vi "AB_820_850_Project_Source.vi"(6 "dataForPrevious":T1, 7 "action":T7, 8 "error in (no error)":errorcluster, 9 "index in":i32, 10 "dataSource in":T6, 11 "buildObject":T4) -> (0 "error out":errorcluster, 1 "index out":i32, 2 "dataSource out":T6, 3 "buildObject out":T4)   [LabVIEW 2020]
doc: "Reads and writes the data to the object property bag."
uses:
  <resource>/Framework/Providers/API/ItemRef.ctl
  <vilib>/AppBuilder/AB_Source_Inclusion.ctl
  <vilib>/AppBuilder/RW_Project/AB_RW_Project_PropBag_Action.ctl
  <vilib>/AppBuilder/RW_Project/AB_RW_Project_Source_Data_for_Previous.ctl
  <vilib>/AppBuilder/AB_BuildType.ctl
  <vilib>/Utility/lvfile.llb/LVFileType.ctl
  <vilib>/AppBuilder/AB_Source_Property_WindowBehavior.ctl
  <vilib>/Utility/lvfile.llb/NI_FileType.lvlib
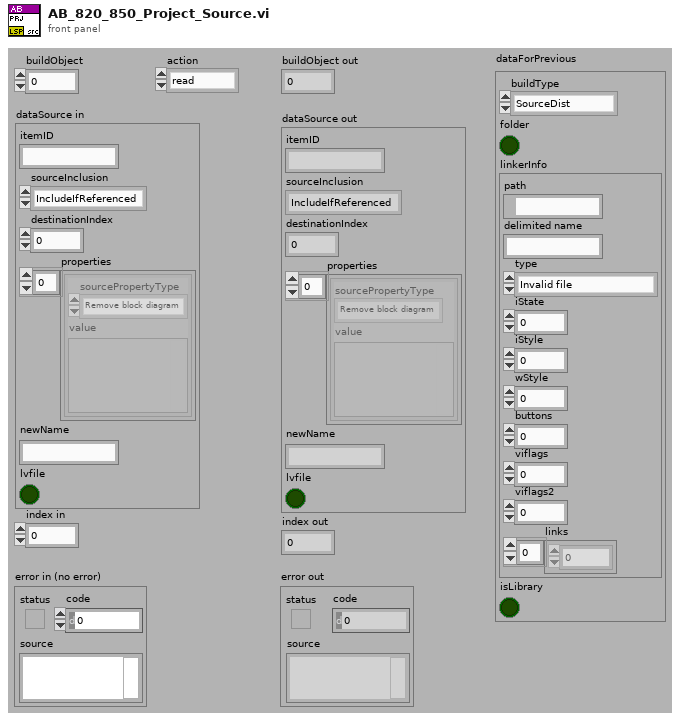
[diagram p1: front panel]
types:
  T1 = typedef "AB_RW_Project_Source_Data_for_Previous.ctl" = cluster{"buildType":T2, "folder":bool, "linkerInfo":cluster{"path":path, "delimited name":string, "type":T3, "iState":u32, "iStyle":u16, "wStyle":u16, "buttons":u16, "viflags":u32, "viflags2":u32, "links":u32[]}, "isLibrary":bool}
  T2 = typedef "AB_BuildType.ctl" = enum16{"SourceDist", "EXE", "DLL", "RTExe"}
  T3 = typedef "NI_FileType.lvlib/LVFileType.ctl" = enum32{"Invalid file", "Unknown type", "Instrument", "Control", "Polymorphic VI", "Project", "Library", "LVClass", "XControl", "XNode", "Shared library", ".NET assembly", "ActiveX interface", "CIN", "Run-time menu", "Palette menu", "Help file", "LLB", "XNode Edit Dependency", "Class Private Data Control", "Statechart", "MathScript .m file", "Ladder Diagram", "LVLibp", "XNode Build Dependency"}
  T4 = typedef "ItemRef.ctl" = u64
  T5 = typedef "AB_Source_Inclusion.ctl" = enum16{"IncludeIfReferenced", "Include", "Exclude", "TopLevel"}
  T6 = cluster{"itemID":string, "sourceInclusion":T5, "destinationIndex":i32, "properties":cluster{"sourcePropertyType":enum16{"Remove block diagram", "Remove front panel", "Password", "Window has title bar", "Show menu bar", "Show vertical scroll bar", "Show horizontal scroll bar", "Show toolbar", "Show Abort button", "Show fp when called", "Window behavior", "Allow user to close window", "Window run-time position", "Run when opened", "Allow debugging", "Auto error handling"}, "value":variant}[], "newName":string, "lvfile":bool}
  T7 = typedef "AB_RW_Project_PropBag_Action.ctl" = enum16{"read", "write", "clear", "readPrevious", "writePrevious", "clearPrevious"}
  T8 = cluster{"sourcePropertyType":enum16{"Remove block diagram", "Remove front panel", "Password", "Window has title bar", "Show menu bar", "Show vertical scroll bar", "Show horizontal scroll bar", "Show toolbar", "Show Abort button", "Show fp when called", "Window behavior", "Allow user to close window", "Window run-time position", "Run when opened", "Allow debugging", "Auto error handling"}, "value":variant}
  T9 = typedef "AB_Source_Property_WindowBehavior.ctl" = enum16{"Default", "Floating", "Modal"}
  T10 = cluster{"sourcePropertyType":enum16{"Remove block diagram", "Remove front panel", "Password", "Window has title bar", "Show menu bar", "Show vertical scroll bar", "Show horizontal scroll bar", "Show toolbar", "Show Abort button", "Show fp when called", "Window behavior", "Allow user to close window", "Window run-time position", "Run when opened", "Allow debugging", "Auto error handling"}, "value":variant}[]
  T11 = enum16{"Remove block diagram", "Remove front panel", "Password", "Window has title bar", "Show menu bar", "Show vertical scroll bar", "Show horizontal scroll bar", "Show toolbar", "Show Abort button", "Show fp when called", "Window behavior", "Allow user to close window", "Window run-time position", "Run when opened", "Allow debugging", "Auto error handling"}
  T12 = enum16{"Remove debugging", "Remove diagram", "Remove panel", "Show panel when called", "Run when opened", "Show abort button", "Window is modal", "Allow user to close window", "Window has title bar", "Show menu bar", "Show tool bar when running", "Show scroll bars", "Auto-center", "Size to entire screen", "Automatic error handling"}
  T13 = cluster{"applyInclusion":bool, "applyDestination":bool, "applyProperties":bool, "applyPassword":bool, "applyPrefix":bool, "applySaveSetttings":bool}
  T14 = cluster{"sourcePropertyType":enum16{"Remove block diagram", "Remove front panel", "Password", "Window has title bar", "Show menu bar", "Show vertical scroll bar", "Show horizontal scroll bar", "Show toolbar", "Show Abort button", "Show fp when called", "Window behavior", "Allow user to close window", "Window run-time position", "Run when opened", "Allow debugging", "Auto error handling"}, "Value":string}
  T15 = cluster{"sourcePropertyType":enum16{"Remove block diagram", "Remove front panel", "Password", "Window has title bar", "Show menu bar", "Show vertical scroll bar", "Show horizontal scroll bar", "Show toolbar", "Show Abort button", "Show fp when called", "Window behavior", "Allow user to close window", "Window run-time position", "Run when opened", "Allow debugging", "Auto error handling"}, string}
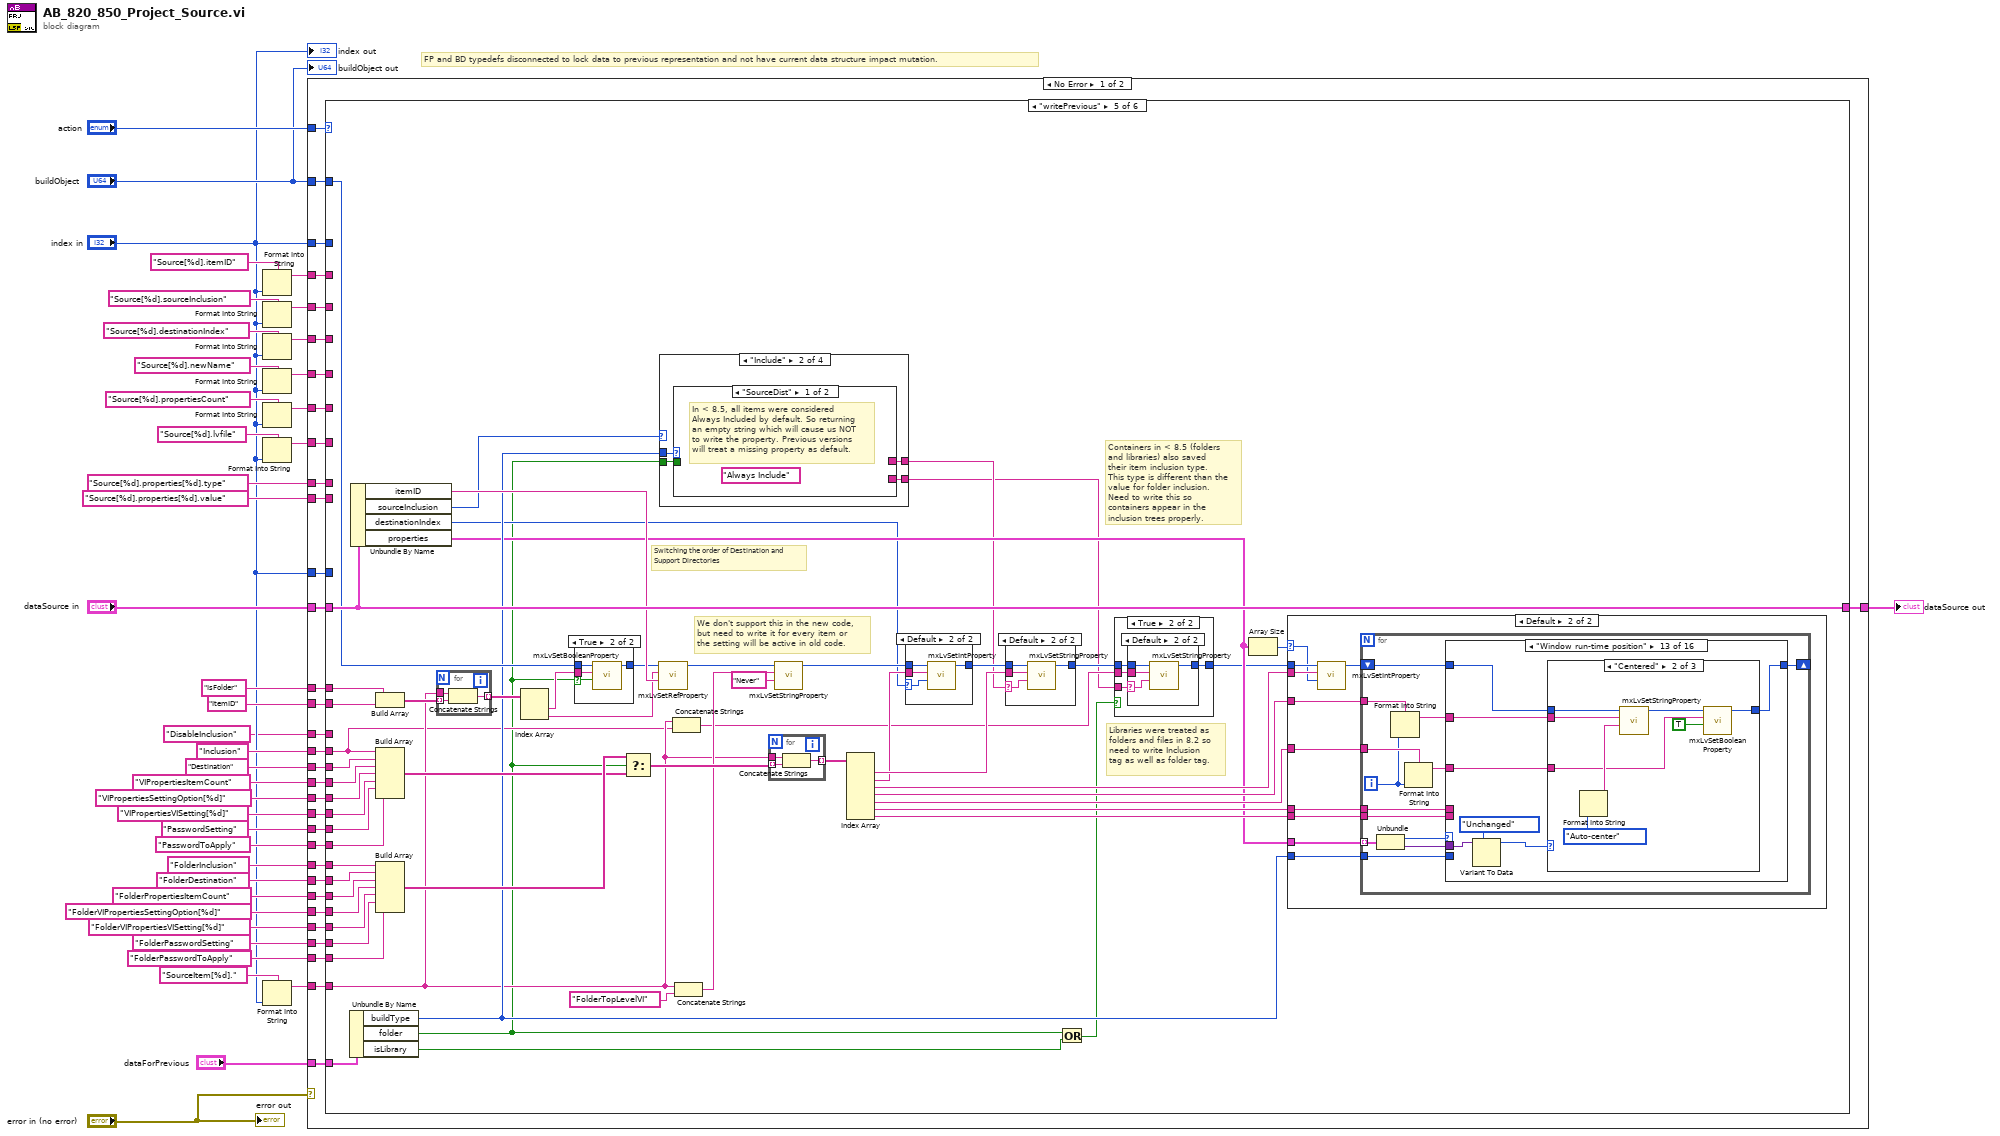
[diagram p0: block diagram]
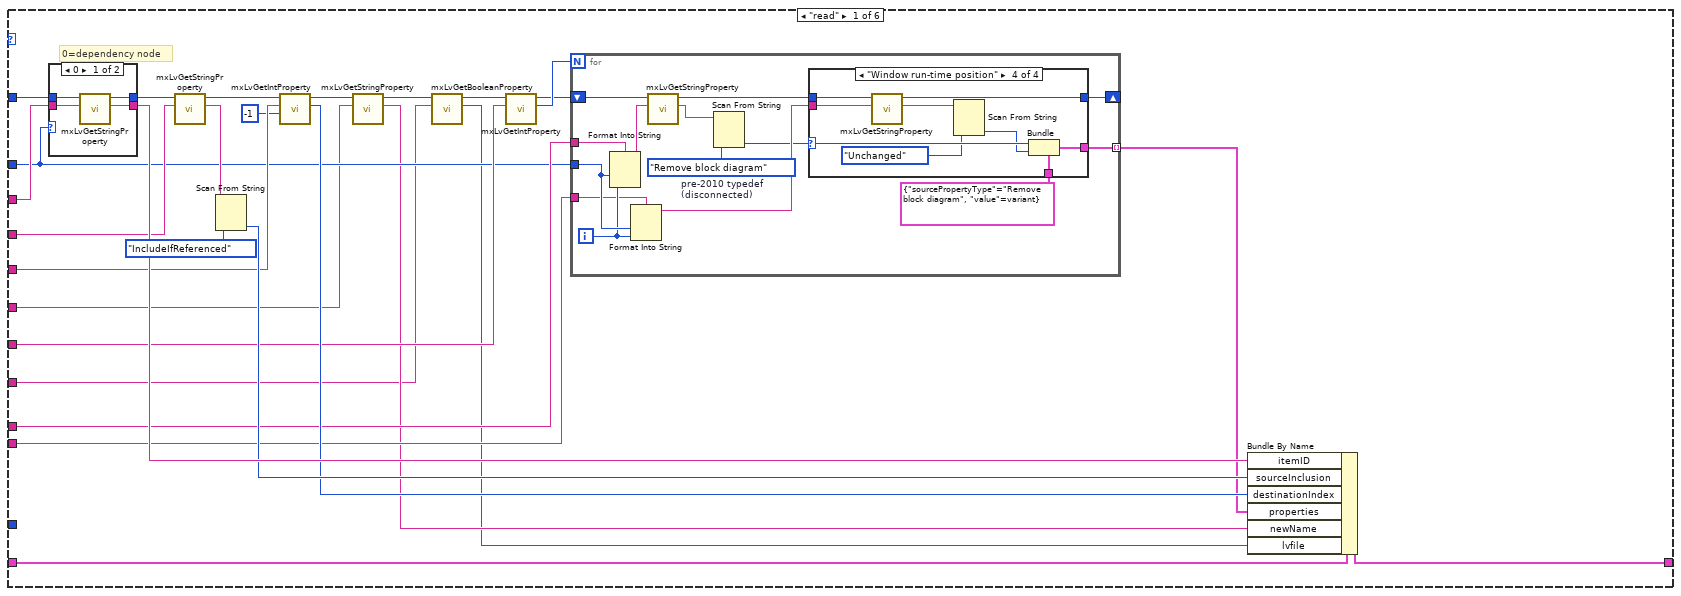
[diagram p2: hidden frame]
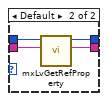
[diagram p3: hidden frame]
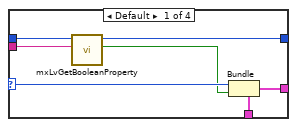
[diagram p4: hidden frame]
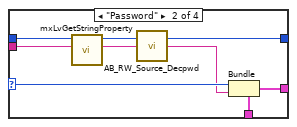
[diagram p5: hidden frame]
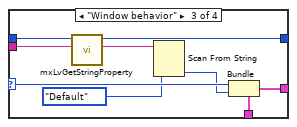
[diagram p6: hidden frame]
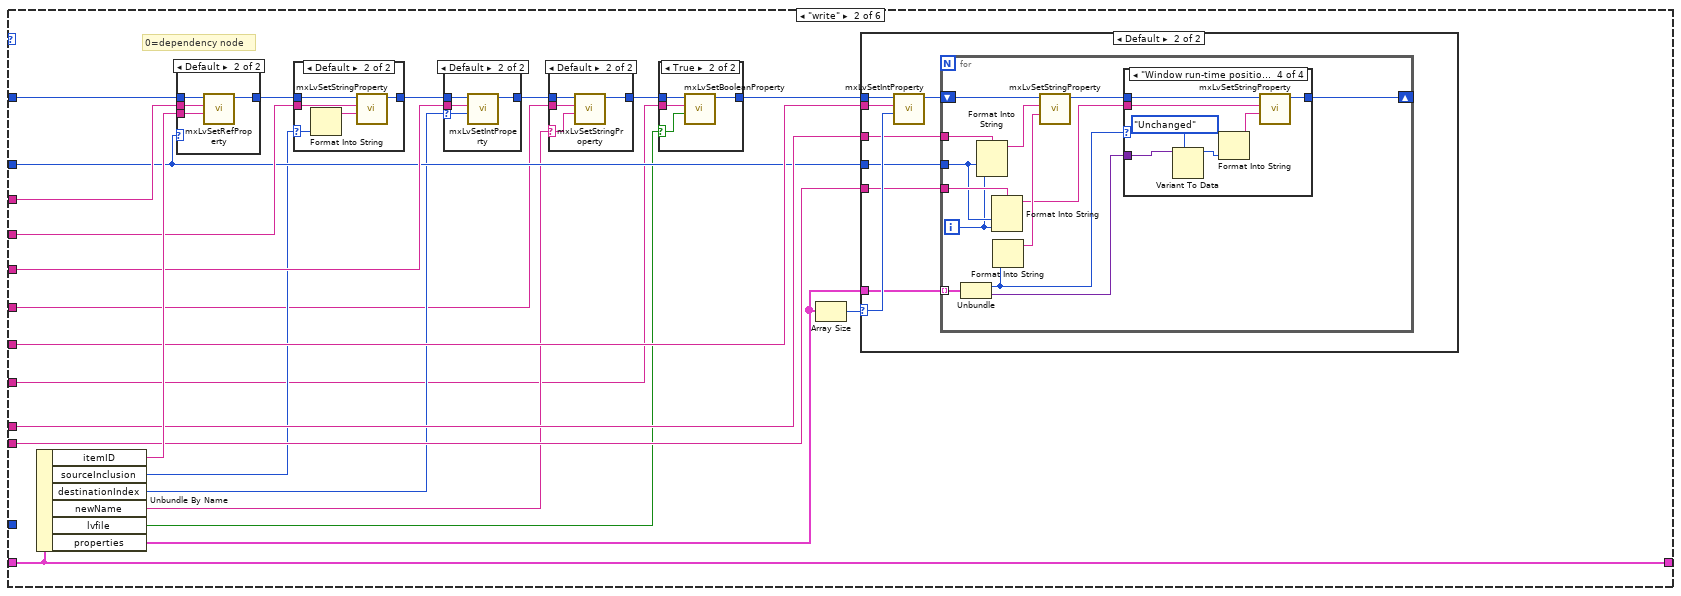
[diagram p7: hidden frame]
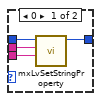
[diagram p12: hidden frame]
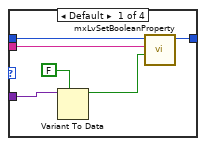
[diagram p14: hidden frame]
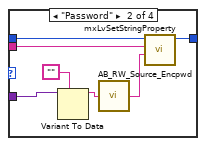
[diagram p15: hidden frame]
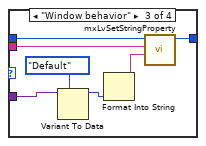
[diagram p16: hidden frame]
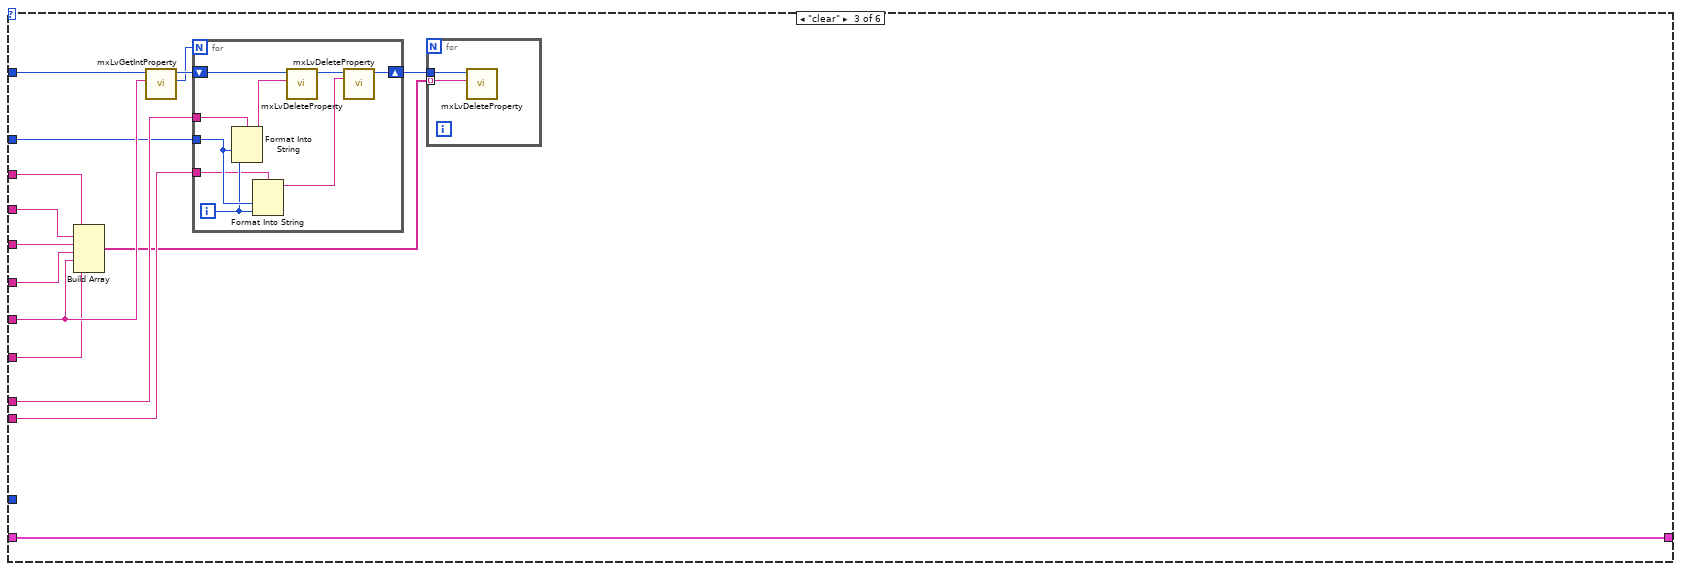
[diagram p17: hidden frame]
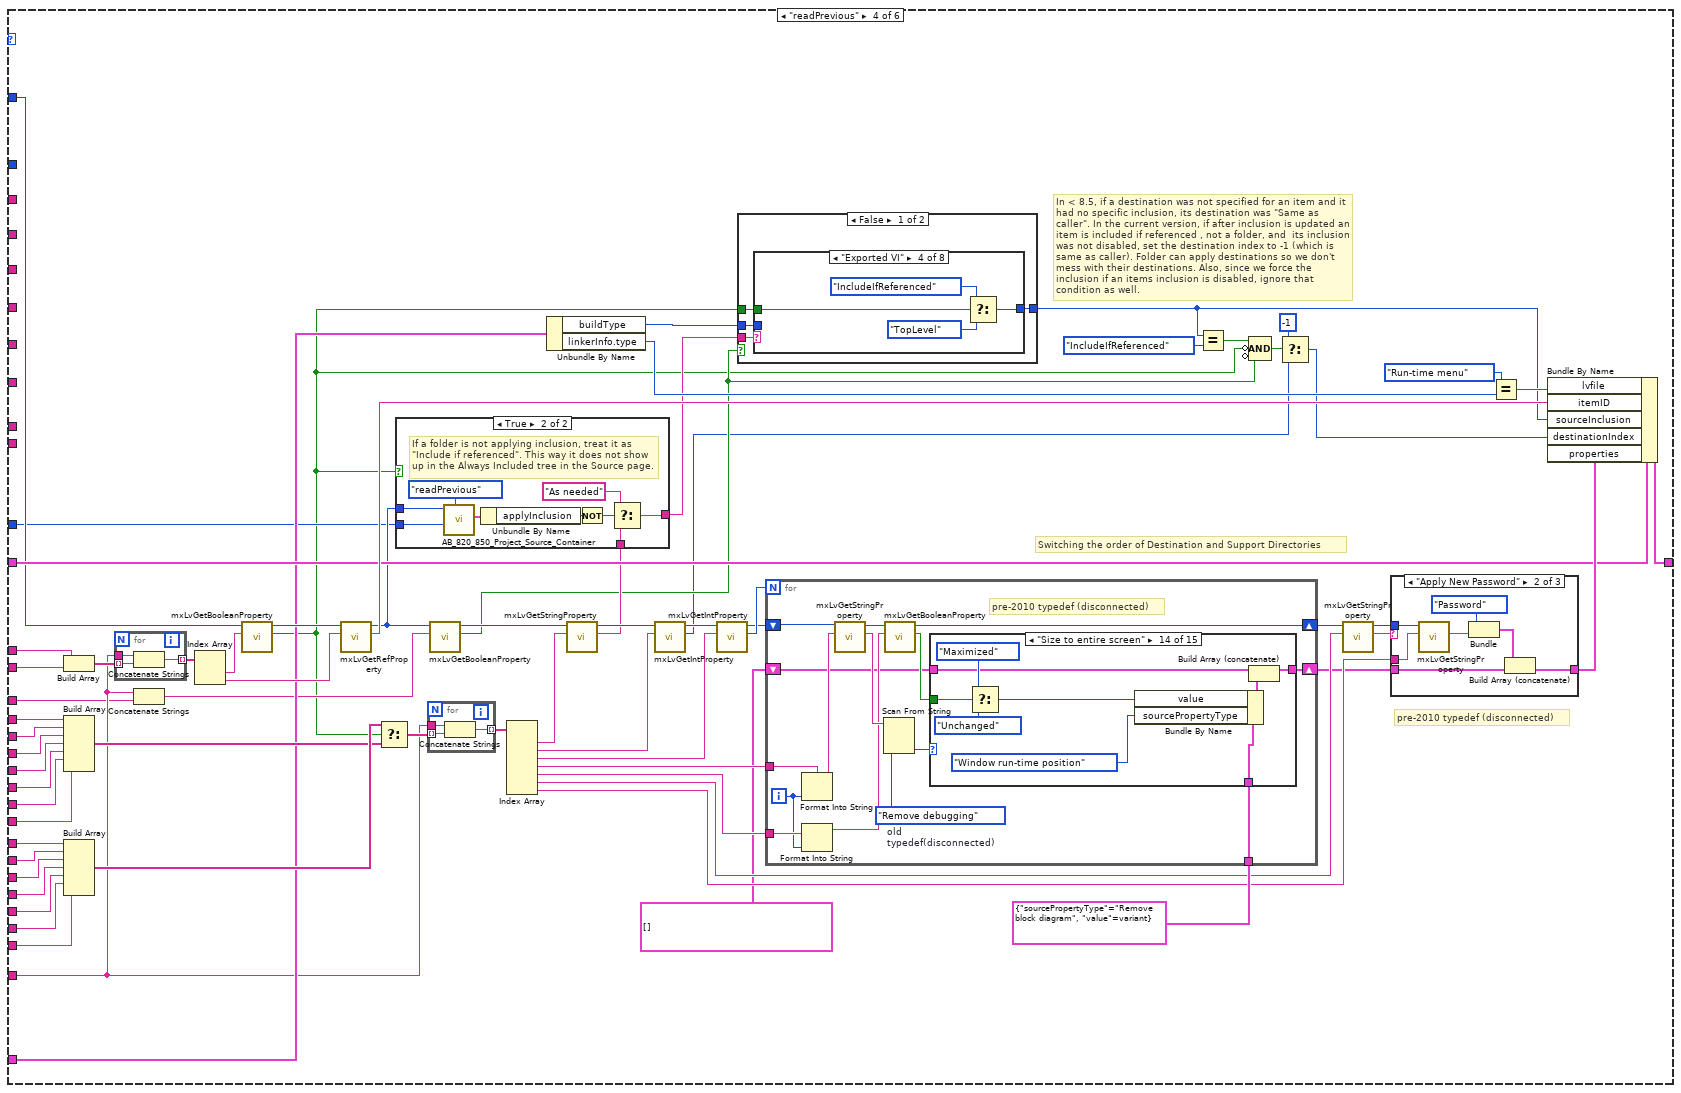
[diagram p18: hidden frame]
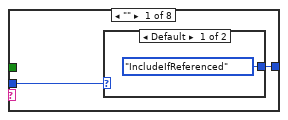
[diagram p20: hidden frame]
diagram:
  # "FP and BD typedefs disconnected to lock data to previous representation and not have current data structure impact mutation."
  n1 = Format Into String(format string="Source[%d].itemID", "index in") -> (resulting string=w37:string)  [unwired: 2 in, 1 out]
  n2 = Format Into String(format string="Source[%d].sourceInclusion", "index in") -> (resulting string=w33:string)  [unwired: 2 in, 1 out]
  n3 = Format Into String(format string="Source[%d].destinationIndex", "index in") -> (resulting string=w32:string)  [unwired: 2 in, 1 out]
  n4 = Format Into String(format string="Source[%d].newName", "index in") -> (resulting string=w5:string)  [unwired: 2 in, 1 out]
  n5 = Format Into String(format string="Source[%d].propertiesCount", "index in") -> (resulting string=w31:string)  [unwired: 2 in, 1 out]
  n6 = Format Into String(format string="Source[%d].lvfile", "index in") -> (resulting string=w3:string)  [unwired: 2 in, 1 out]
  n7 = Format Into String(format string="SourceItem[%d].", "index in") -> (resulting string=w24:string)  [unwired: 2 in, 1 out]
  n8 = case shown="No Error" "error in (no error)" {
    tunnel: "action" -> [w73 _]
    tunnel: "dataSource in" -> [w72 w901]
    tunnel: w37 -> [w71 _]
    tunnel: w33 -> [w70 _]
    tunnel: w32 -> [w69 _]
    tunnel: w31 -> [w68 _]
    tunnel: "Source[%d].properties[%d].type" -> [w67 _]
    tunnel: "index in" -> [w66 _]
    tunnel: "Source[%d].properties[%d].value" -> [w65 _]
    tunnel: [w64 w901] -> w28
    tunnel: "buildObject" -> [w63 _]
    tunnel: w24 -> [w62 _]
    tunnel: "Inclusion" -> [w61 _]
    tunnel: "Destination" -> [w60 _]
    tunnel: "VIPropertiesItemCount" -> [w59 _]
    tunnel: "VIPropertiesSettingOption[%d]" -> [w58 _]
    tunnel: "VIPropertiesVISetting[%d]" -> [w57 _]
    tunnel: "PasswordSetting" -> [w56 _]
    tunnel: "PasswordToApply" -> [w55 _]
    tunnel: "FolderInclusion" -> [w54 _]
    tunnel: "FolderDestination" -> [w53 _]
    tunnel: "FolderPropertiesItemCount" -> [w52 _]
    tunnel: "FolderVIPropertiesSettingOption[%d]" -> [w51 _]
    tunnel: "FolderVIPropertiesVISetting[%d]" -> [w50 _]
    tunnel: "FolderPasswordSetting" -> [w49 _]
    tunnel: "FolderPasswordToApply" -> [w48 _]
    tunnel: "ItemID" -> [w47 _]
    tunnel: "IsFolder" -> [w46 _]
    tunnel: "dataForPrevious" -> [w45 _]
    tunnel: w5 -> [w44 _]
    tunnel: w3 -> [w43 _]
    tunnel: "index in" -> [w42 _]
    tunnel: "DisableInclusion" -> [w41 _]
    frame No Error {
      n9 = case shown="\"writePrevious\"" w73 {
        tunnel: w63 -> [w101 w178 w267 w295 w547 w865]
        tunnel: w72 -> [w100 w179 w271 w310 w572 w879]
        tunnel: w71 -> [w98 w177 w270 _ _ _]
        tunnel: w70 -> [w96 w174 w269 _ _ _]
        tunnel: w69 -> [w91 w172 w268 _ _ _]
        tunnel: w68 -> [w89 w169 w265 _ _ _]
        tunnel: w67 -> [w87 w168 w263 _ _ _]
        tunnel: w66 -> [w82 w166 w261 _ _ _]
        tunnel: w65 -> [w85 w167 w262 _ _ _]
        tunnel: [w83 w179 w271 w351 w572 w879] -> w64
        tunnel: w62 -> [_ _ _ w300 w523 w854]
        tunnel: w61 -> [_ _ _ w341 w522 w875]
        tunnel: w60 -> [_ _ _ w340 w564 w874]
        tunnel: w59 -> [_ _ _ w339 w563 w862]
        tunnel: w58 -> [_ _ _ w338 w562 w861]
        tunnel: w57 -> [_ _ _ w337 w561 w858]
        tunnel: w56 -> [_ _ _ w336 w560 w873]
        tunnel: w55 -> [_ _ _ w335 w559 w872]
        tunnel: w54 -> [_ _ _ w334 w558 w871]
        tunnel: w53 -> [_ _ _ w333 w557 w870]
        tunnel: w52 -> [_ _ _ w332 w556 w859]
        tunnel: w51 -> [_ _ _ w331 w555 w856]
        tunnel: w50 -> [_ _ _ w330 w554 w855]
        tunnel: w49 -> [_ _ _ w329 w553 w869]
        tunnel: w48 -> [_ _ _ w328 w552 w868]
        tunnel: w47 -> [_ _ _ w327 w565 w847]
        tunnel: w46 -> [_ _ _ w326 w566 w846]
        tunnel: w45 -> [_ _ _ w305 w549 _]
        tunnel: w44 -> [w79 w161 w258 _ _ _]
        tunnel: w43 -> [w77 w158 w257 _ _ _]
        tunnel: w42 -> [_ _ _ w292 _ _]
        tunnel: w41 -> [_ _ _ w299 _ _]
        frame "read" {
          # "0=dependency node"
          n10 = case shown="0" w82 {
            tunnel: w101 -> [w105 w109]
            tunnel: [w102 w108] -> w99
            tunnel: w98 -> [w103 w107]
            tunnel: [w104 w106] -> w97
            frame 0 {
              n11 = call <resource>:"mxLvGetStringProperty.vi"("Tag"=w103, "Item"=w105) -> ("Value"=w102:string, "Item"=w104:T4)  [unwired: 7 in, 1 out]
            }
            frame Default {
              n12 = call <resource>:"mxLvGetRefProperty.vi"("Tag"=w107, "Item"=w109) -> ("Value"=w108:string, "Item"=w106:T4)  [unwired: 7 in, 1 out]
            }
          }
          n13 = call <resource>:"mxLvGetStringProperty.vi"("Tag"=w96, "Item"=w97) -> ("Value"=w95:string, "Item"=w92:T4)  [unwired: 7 in, 1 out]
          n14 = Scan From String(input string=w95, default 1=AB_Source_Inclusion."IncludeIfReferenced" ("sourceInclusion")) -> (output 1=w93:T5)  [unwired: 3 in, 3 out]
          n15 = call <resource>:"mxLvGetIntProperty.vi"("Default Value (0)"=-1, "Tag"=w91, "Item"=w92) -> ("Value"=w90:i32, "Item"=w80:T4)  [unwired: 6 in, 1 out]
          n16 = call <resource>:"mxLvGetStringProperty.vi"("Tag"=w79, "Item"=w80) -> ("Value"=w78:string, "Item"=w75:T4)  [unwired: 7 in, 1 out]
          n17 = call <resource>:"mxLvGetBooleanProperty.vi"("Tag"=w77, "Item"=w75) -> ("Value"=w76:bool, "Item"=w74:T4)  [unwired: 7 in, 1 out]
          n18 = call <resource>:"mxLvGetIntProperty.vi"("Tag"=w89, "Item"=w74) -> ("Value"=w88:i32, "Item"=w86:T4)  [unwired: 7 in, 1 out]
          n19 = for {
            N: w88 -> [_]
            tunnel: w87 -> [w123]
            tunnel: w82 -> [w117]
            shift-right: [w113] -> _
            shift-left: w86 -> [w122]
            tunnel: w85 -> [w115]
            tunnel: [w111] -> w84 mode=indexing
            i -> [w116]
            w120 = T11."Remove block diagram"  # pre-2010 typedef (disconnected)
            n20 = Format Into String(format string=w123, w117, w116) -> (resulting string=w121:string)  [unwired: 2 in, 1 out]
            n21 = Format Into String(format string=w115, w117, w116) -> (resulting string=w114:string)  [unwired: 2 in, 1 out]
            n22 = call <resource>:"mxLvGetStringProperty.vi"("Tag"=w121, "Item"=w122) -> ("Value"=w119:string, "Item"=w118:T4)  [unwired: 7 in, 1 out]
            n23 = Scan From String(input string=w119, default 1=w120) -> (output 1=w112:T11)  [unwired: 3 in, 3 out]
            n24 = case shown="\"Window run-time position\"" w112 {
              selector: w112 -> [w127 w135 w144 w153]
              tunnel: w118 -> [w130 w138 w147 w156]
              tunnel: w114 -> [w129 w136 w145 w154]
              tunnel: [w128 w137 w146 w155] -> w113
              tunnel: [w125 w133 w142 w151] -> w111
              tunnel: T8 {"sourcePropertyType"=enum."Remove block diagram", "value"=variant} ("fileProperties") -> [w124 w134 w143 w152]
              frame Default {
                n25 = call <resource>:"mxLvGetBooleanProperty.vi"("Tag"=w129, "Item"=w130) -> ("Value"=w126:bool, "Item"=w128:T4)  [unwired: 7 in, 1 out]
                n26 = Bundle(cluster=w124, "sourcePropertyType"=w127, "value"=w126) -> (w125:T8)
              }
              frame "Password" {
                n27 = call <resource>:"mxLvGetStringProperty.vi"("Tag"=w136, "Item"=w138) -> ("Value"=w132:string, "Item"=w137:T4)  [unwired: 7 in, 1 out]
                n28 = call <vilib>:"AB_RW_Source_Decpwd.vi"("input string"=w132) -> ("output string"=w131:string)
                n29 = Bundle(cluster=w134, "sourcePropertyType"=w135, "value"=w131) -> (w133:T8)
              }
              frame "Window behavior" {
                n30 = call <resource>:"mxLvGetStringProperty.vi"("Tag"=w145, "Item"=w147) -> ("Value"=w141:string, "Item"=w146:T4)  [unwired: 7 in, 1 out]
                n31 = Scan From String(input string=w141, default 1=AB_Source_Property_WindowBehavior."Default" ("windowBehavior")) -> (output 1=w140:T9)  [unwired: 3 in, 3 out]
                n32 = Bundle(cluster=w143, "sourcePropertyType"=w144, "value"=w140) -> (w142:T8)
              }
              frame "Window run-time position" {
                n33 = call <resource>:"mxLvGetStringProperty.vi"("Tag"=w154, "Item"=w156) -> ("Value"=w150:string, "Item"=w155:T4)  [unwired: 7 in, 1 out]
                n34 = Scan From String(input string=w150, default 1=enum16{"Unchanged", "Centered", "Maximized"}."Unchanged" ("windowRunTimePosition")) -> (output 1=w149:enum16{"Unchanged", "Centered", "Maximized"})  [unwired: 3 in, 3 out]
                n35 = Bundle(cluster=w152, "sourcePropertyType"=w153, "value"=w149) -> (w151:T8)
              }
            }
          }
          n36 = Bundle By Name(cluster=w100, "itemID"=w99, "sourceInclusion"=w93, "destinationIndex"=w90, "properties"=w84, "newName"=w78, "lvfile"=w76) -> (w83:T6)
        }
        frame "write" {
          # "0=dependency node"
          n37 = Unbundle By Name(w179) -> ("itemID"=w176:string, "sourceInclusion"=w165:T5, "destinationIndex"=w164:i32, "newName"=w162:string, "lvfile"=w157:bool, "properties"=w171:T10)
          n38 = case shown="Default" w166 {
            tunnel: w178 -> [w204 w208]
            tunnel: w177 -> [w202 w207]
            tunnel: w176 -> [w201 w206]
            tunnel: [w203 w205] -> w175
            frame 0 {
              n39 = call <resource>:"mxLvSetStringProperty.vi"("Value (\"\")"=w201, "Tag"=w202, "Item"=w204) -> ("Item"=w203:T4)  [unwired: 7 in, 1 out]
            }
            frame Default {
              n40 = call <resource>:"mxLvSetRefProperty.vi"("Value (\"\")"=w206, "Tag"=w207, "Item"=w208) -> ("Item"=w205:T4)  [unwired: 7 in, 1 out]
            }
          }
          n41 = case shown="Default" w165 {
            selector: w165 -> [_ w196]
            tunnel: w175 -> [w195 w200]
            tunnel: w174 -> [_ w198]
            tunnel: [w195 w197] -> w173
            frame "IncludeIfReferenced" {
            }
            frame Default {
              n42 = Format Into String(w196) -> (resulting string=w199:string)  [unwired: 3 in, 1 out]
              n43 = call <resource>:"mxLvSetStringProperty.vi"("Value (\"\")"=w199, "Tag"=w198, "Item"=w200) -> ("Item"=w197:T4)  [unwired: 7 in, 1 out]
            }
          }
          n44 = case shown="Default" w164 {
            selector: w164 -> [_ w191]
            tunnel: w173 -> [w190 w194]
            tunnel: w172 -> [_ w193]
            tunnel: [w190 w192] -> w163
            frame -1 {
            }
            frame Default {
              n45 = call <resource>:"mxLvSetIntProperty.vi"("Value (0)"=w191, "Tag"=w193, "Item"=w194) -> ("Item"=w192:T4)  [unwired: 7 in, 1 out]
            }
          }
          n46 = case shown="Default" w162 {
            selector: w162 -> [_ w186]
            tunnel: w163 -> [w185 w189]
            tunnel: w161 -> [_ w188]
            tunnel: [w185 w187] -> w160
            frame "" {
            }
            frame Default {
              n47 = call <resource>:"mxLvSetStringProperty.vi"("Value (\"\")"=w186, "Tag"=w188, "Item"=w189) -> ("Item"=w187:T4)  [unwired: 7 in, 1 out]
            }
          }
          n48 = case shown="True" w157 {
            selector: w157 -> [_ w181]
            tunnel: w160 -> [w180 w184]
            tunnel: w158 -> [_ w183]
            tunnel: [w180 w182] -> w159
            frame False {
            }
            frame True {
              n49 = call <resource>:"mxLvSetBooleanProperty.vi"("Value (F)"=w181, "Tag"=w183, "Item"=w184) -> ("Item"=w182:T4)  [unwired: 7 in, 1 out]
            }
          }
          n50 = Array Size(array=w171) -> (size(s)=w170:i32)
          n51 = case shown="Default" w170 {
            selector: w170 -> [_ w214]
            tunnel: w171 -> [_ w212]
            tunnel: w169 -> [_ w216]
            tunnel: w159 -> [_ w215]
            tunnel: w168 -> [_ w211]
            tunnel: w166 -> [_ w210]
            tunnel: w167 -> [_ w209]
            frame 0 {
            }
            frame Default {
              n52 = call <resource>:"mxLvSetIntProperty.vi"("Value (0)"=w214, "Tag"=w216, "Item"=w215) -> ("Item"=w213:T4)  [unwired: 7 in, 1 out]
              n53 = for {
                shift-right: [w219] -> _
                shift-left: w213 -> [w229]
                tunnel: w212 -> [w228] mode=indexing
                tunnel: w211 -> [w227]
                tunnel: w210 -> [w223]
                tunnel: w209 -> [w224]
                i -> [w222]
                n54 = Unbundle(w228) -> ("sourcePropertyType"=w221:T11, "value"=w217:variant)
                n55 = Format Into String(format string=w227, w223, w222) -> (resulting string=w226:string)  [unwired: 2 in, 1 out]
                n56 = Format Into String(format string=w224, w223, w222) -> (resulting string=w218:string)  [unwired: 2 in, 1 out]
                n57 = Format Into String(w221) -> (resulting string=w225:string)  [unwired: 3 in, 1 out]
                n58 = call <resource>:"mxLvSetStringProperty.vi"("Value (\"\")"=w225, "Tag"=w226, "Item"=w229) -> ("Item"=w220:T4)  [unwired: 7 in, 1 out]
                n59 = case shown="\"Window run-time position\"" w221 {
                  tunnel: w220 -> [w235 w240 w248 w255]
                  tunnel: [w234 w239 w247 w254] -> w219
                  tunnel: w218 -> [w233 w238 w246 w253]
                  tunnel: w217 -> [w231 w242 w249 w256]
                  frame Default {
                    n60 = Variant To Data(type=FALSE, Variant=w231) -> (data=w230:bool)  [unwired: 1 in, 1 out]
                    n61 = call <resource>:"mxLvSetBooleanProperty.vi"("Value (F)"=w230, "Tag"=w233, "Item"=w235) -> ("Item"=w234:T4)  [unwired: 7 in, 1 out]
                  }
                  frame "Password" {
                    n62 = Variant To Data(type="", Variant=w242) -> (data=w237:string)  [unwired: 1 in, 1 out]
                    n63 = call <vilib>:"AB_RW_Source_Encpwd.vi"("input String"=w237) -> ("output String"=w236:string)  [unwired: 1 in]
                    n64 = call <resource>:"mxLvSetStringProperty.vi"("Value (\"\")"=w236, "Tag"=w238, "Item"=w240) -> ("Item"=w239:T4)  [unwired: 7 in, 1 out]
                  }
                  frame "Window behavior" {
                    n65 = Variant To Data(type=AB_Source_Property_WindowBehavior."Default" ("windowBehavior"), Variant=w249) -> (data=w244:T9)  [unwired: 1 in, 1 out]
                    n66 = Format Into String(w244) -> (resulting string=w243:string)  [unwired: 3 in, 1 out]
                    n67 = call <resource>:"mxLvSetStringProperty.vi"("Value (\"\")"=w243, "Tag"=w246, "Item"=w248) -> ("Item"=w247:T4)  [unwired: 7 in, 1 out]
                  }
                  frame "Window run-time position" {
                    n68 = Variant To Data(type=enum16{"Unchanged", "Centered", "Maximized"}."Unchanged" ("windowRunTimePosition"), Variant=w256) -> (data=w252:enum16{"Unchanged", "Centered", "Maximized"})  [unwired: 1 in, 1 out]
                    n69 = Format Into String(w252) -> (resulting string=w251:string)  [unwired: 3 in, 1 out]
                    n70 = call <resource>:"mxLvSetStringProperty.vi"("Value (\"\")"=w251, "Tag"=w253, "Item"=w255) -> ("Item"=w254:T4)  [unwired: 7 in, 1 out]
                  }
                }
              }
            }
          }
        }
        frame "clear" {
          n71 = Build Array(w270, w269, w268, w258, w265, w257) -> (w259:string[])
          n72 = call <resource>:"mxLvGetIntProperty.vi"("Tag"=w265, "Item"=w267) -> ("Value"=w264:i32, "Item"=w266:T4)  [unwired: 7 in, 1 out]
          n73 = for {
            N: w264 -> [_]
            tunnel: w263 -> [w282]
            tunnel: w261 -> [w281]
            shift-right: [w276] -> w260
            shift-left: w266 -> [w278]
            tunnel: w262 -> [w279]
            i -> [w280]
            n74 = Format Into String(format string=w282, w281, w280) -> (resulting string=w275:string)  [unwired: 2 in, 1 out]
            n75 = Format Into String(format string=w279, w281, w280) -> (resulting string=w274:string)  [unwired: 2 in, 1 out]
            n76 = call <resource>:"mxLvDeleteProperty.vi"("Tag"=w275, "Item"=w278) -> ("Item"=w277:T4)  [unwired: 8 in, 1 out]
            n77 = call <resource>:"mxLvDeleteProperty.vi"("Tag"=w274, "Item"=w277) -> ("Item"=w276:T4)  [unwired: 8 in, 1 out]
          }
          n78 = for {
            tunnel: w260 -> [w273]
            tunnel: w259 -> [w272] mode=indexing
            n79 = call <resource>:"mxLvDeleteProperty.vi"("Tag"=w272, "Item"=w273) -> ()  [unwired: 8 in, 2 out]
          }
        }
        frame "readPrevious" {
          # "pre-2010 typedef (disconnected)"
          # "In < 8.5, if a destination was not specified for an item and it had no specific inclusion, its destination was \"Same as caller\". In the current version, if after inclusion is updated an item is included if referenced , not a folder, and  its inclusion was not disabled, set the destination index to -1 (which is same as caller). Folder can apply destinations so we don't mess with their destinations. Also, since we force the inclusion if an items inclusion is disabled, ignore that condition as well."
          # "Switching the order of Destination and Support Directories"
          n80 = Build Array(w326, w327) -> (w325:string[])
          n81 = Build Array(w341, w340, w339, w338, w337, w336, w335) -> (w308:string[])
          n82 = Build Array(w334, w333, w332, w331, w330, w329, w328) -> (w309:string[])
          n83 = for {
            tunnel: w300 -> [w386]
            tunnel: w325 -> [w385] mode=indexing
            tunnel: [w384] -> w323 mode=indexing
            n84 = Concatenate Strings(w386, w385) -> (w384:string)
          }
          n85 = Concatenate Strings(w300, w299) -> (w298:string)
          n86 = Index Array(array=w323) -> (element #1=w322:string, element #2=w321:string)  [unwired: 2 in]
          n87 = call <resource>:"mxLvGetBooleanProperty.vi"("Tag"=w322, "Item"=w295) -> ("Value"=w287:bool, "Item"=w343:T4)  [unwired: 7 in, 1 out]
          n88 = call <resource>:"mxLvGetRefProperty.vi"("Tag"=w321, "Item"=w343) -> ("Value"=w342:string, "Item"=w294:T4)  [unwired: 7 in, 1 out]
          n89 = Select(t=w309, s=w287, f=w308) -> (s? t:f=w324:string[])
          n90 = for {
            tunnel: w300 -> [w383]
            tunnel: w324 -> [w382] mode=indexing
            tunnel: [w381] -> w320 mode=indexing
            n91 = Concatenate Strings(w383, w382) -> (w381:string)
          }
          n92 = call <resource>:"mxLvGetBooleanProperty.vi"("Tag"=w298, "Item"=w294) -> ("Value"=w288:bool, "Item"=w293:T4)  [unwired: 7 in, 1 out]
          n93 = Index Array(array=w320) -> (element #1=w319:string, element #2=w317:string, element #3=w315:string, element #4=w318:string, element #5=w311:string, element #6=w314:string, element #7=w313:string)  [unwired: 7 in]
          n94 = Unbundle By Name(w305) -> ("buildType"=w304:T2, "linkerInfo.type"=w302:T3)
          n95 = call <resource>:"mxLvGetStringProperty.vi"("Tag"=w319, "Item"=w293) -> ("Value"=w297:string, "Item"=w316:T4)  [unwired: 7 in, 1 out]
          n96 = case shown="True" w287 {
            tunnel: w294 -> [_ w358]
            tunnel: w297 -> [w352 w354]
            tunnel: [w352 w357] -> w296
            tunnel: w292 -> [_ w356]
            frame False {
            }
            frame True {
              # "If a folder is not applying inclusion, treat it as \"Include if referenced\". This way it does not show up in the Always Included tree in the Source page."
              n97 = call <vilib>:"AB_820_850_Project_Source_Container.vi"("action"=AB_RW_Project_PropBag_Action."readPrevious", "index in"=w356, "buildObject"=w358) -> ("dataSource out"=w360:T13)  [unwired: 5 in, 3 out]
              n98 = Unbundle By Name(w360) -> ("applyInclusion"=w359:bool)
              n99 = Not(x=w359) -> (.not. x?=w355:bool)
              n100 = Select(t="As needed", s=w355, f=w354) -> (s? t:f=w357:string)
            }
          }
          n101 = call <resource>:"mxLvGetIntProperty.vi"("Tag"=w317, "Item"=w316) -> ("Value"=w285:i32, "Item"=w350:T4)  [unwired: 7 in, 1 out]
          n102 = call <resource>:"mxLvGetIntProperty.vi"("Tag"=w315, "Item"=w350) -> ("Value"=w349:i32, "Item"=w312:T4)  [unwired: 7 in, 1 out]
          n103 = case shown="False" w288 {
            tunnel: [w365 AB_Source_Inclusion."IncludeIfReferenced" ("sourceInfo.sourceInclusion")] -> w290
            tunnel: w304 -> [w364 _]
            tunnel: w287 -> [w363 _]
            tunnel: w296 -> [w362 _]
            frame False {
              n104 = case shown="\"Exported VI\"" w362 {
                tunnel: [w367 AB_Source_Inclusion."IncludeIfReferenced" ("sourceInfo.sourceInclusion") AB_Source_Inclusion."TopLevel" ("sourceInfo.sourceInclusion") w372 AB_Source_Inclusion."TopLevel" ("sourceInfo.sourceInclusion") AB_Source_Inclusion."Include" ("sourceInfo.sourceInclusion") AB_Source_Inclusion."Include" ("sourceInfo.sourceInclusion") AB_Source_Inclusion."Exclude" ("sourceInfo.sourceInclusion")] -> w365
                tunnel: w363 -> [_ _ _ w375 _ _ _ _]
                tunnel: w364 -> [w366 _ _ _ _ _ _ _]
                frame "" {
                  n105 = case shown="Default" w366 {
                    tunnel: [AB_Source_Inclusion."IncludeIfReferenced" ("sourceInfo.sourceInclusion") AB_Source_Inclusion."Include" ("sourceInfo.sourceInclusion")] -> w367
                    frame Default {
                    }
                    frame "SourceDist" {
                    }
                  }
                }
                frame "As needed" {
                }
                frame "Startup VI" {
                }
                frame "Exported VI" {
                  n106 = Select(t=AB_Source_Inclusion."IncludeIfReferenced" ("sourceInfo.sourceInclusion"), s=w375, f=AB_Source_Inclusion."TopLevel" ("sourceInfo.sourceInclusion")) -> (s? t:f=w372:T5)
                }
                frame "Top-level VI (for non-VIs, always inclue)" {
                  # "\"Include\" is misspelled but that's the way it was. DON'T CORRECT."
                }
                frame "Always Included", Default {
                }
                frame "Dynamic VI (for non-VIs, always include)" {
                }
                frame "Always Exclude" {
                }
              }
            }
            frame True {
              # "If this item has the DisableInclusion flag set, its parent had set the inclusion in a previous version. So set this item as incluide if referenced. Code downstream will handle the parent applying its inclusion."
            }
          }
          n107 = for {
            N: w349 -> [_]
            tunnel: T8 {"sourcePropertyType"=enum."Remove block diagram", "value"=variant} ("fileProperties") -> [w402]
            tunnel: w318 -> [w410]
            tunnel: w311 -> [w407]
            shift-right: [w411] -> w347
            shift-left: w312 -> [w414]
            shift-right: [w401] -> w307
            shift-left: T10 [] -> [w400]
            i -> [w406]
            w404 = T12."Remove debugging"  # old typedef(disconnected)
            # "pre-2010 typedef (disconnected)"
            n108 = Format Into String(format string=w410, w406) -> (resulting string=w409:string)  [unwired: 2 in, 1 out]
            n109 = Format Into String(format string=w407, w406) -> (resulting string=w408:string)  [unwired: 2 in, 1 out]
            n110 = call <resource>:"mxLvGetStringProperty.vi"("Tag"=w409, "Item"=w414) -> ("Value"=w412:string, "Item"=w413:T4)  [unwired: 7 in, 1 out]
            n111 = Scan From String(input string=w412, default 1=w404) -> (output 1=w405:T12)  [unwired: 3 in, 3 out]
            n112 = call <resource>:"mxLvGetBooleanProperty.vi"("Tag"=w408, "Item"=w413) -> ("Value"=w403:bool, "Item"=w411:T4)  [unwired: 7 in, 1 out]
            n113 = case shown="\"Size to entire screen\"" w405 {
              tunnel: w403 -> [w421 w425 w432 w437 w443 w448 w460 w462 w467 w473 w480 w485 w501 w510 w511]
              tunnel: w402 -> [w419 w422 w428 w434 w440 w447 w454 w461 w469 w475 w479 w487 w493 w502 w513]
              tunnel: [w417 w423 w429 w435 w441 w446 w455 w464 w470 w476 w482 w490 w496 w505 w514] -> w401
              tunnel: w400 -> [w416 w424 w430 w436 w442 w450 w456 w465 w471 w477 w483 w491 w497 w506 w515]
              frame "Remove debugging" {
                n114 = Not(x=w421) -> (.not. x?=w415:bool)
                n115 = Bundle By Name(cluster=w419, "value"=w415, "sourcePropertyType"=T11."Allow debugging") -> (w418:T8)
                n116 = Build Array (concatenate)(w416, w418) -> (w417:T10)
              }
              frame "Remove diagram" {
                n117 = Bundle By Name(cluster=w422, "value"=w425, "sourcePropertyType"=T11."Remove block diagram") -> (w427:T8)
                n118 = Build Array (concatenate)(w424, w427) -> (w423:T10)
              }
              frame "Remove panel" {
                n119 = Bundle By Name(cluster=w428, "value"=w432, "sourcePropertyType"=T11."Remove front panel") -> (w433:T8)
                n120 = Build Array (concatenate)(w430, w433) -> (w429:T10)
              }
              frame "Show panel when called" {
                n121 = Bundle By Name(cluster=w434, "value"=w437, "sourcePropertyType"=T11."Show fp when called") -> (w439:T8)
                n122 = Build Array (concatenate)(w436, w439) -> (w435:T10)
              }
              frame "Run when opened" {
                n123 = Bundle By Name(cluster=w440, "value"=w443, "sourcePropertyType"=T11."Run when opened") -> (w445:T8)
                n124 = Build Array (concatenate)(w442, w445) -> (w441:T10)
              }
              frame "Show abort button" {
                n125 = Bundle By Name(cluster=w447, "value"=w448, "sourcePropertyType"=T11."Show Abort button") -> (w451:T8)
                n126 = Build Array (concatenate)(w450, w451) -> (w446:T10)
              }
              frame "Window is modal" {
                n127 = Select(t=AB_Source_Property_WindowBehavior."Modal" ("windowBehavior"), s=w460, f=AB_Source_Property_WindowBehavior."Default" ("windowBehavior")) -> (s? t:f=w453:T9)
                n128 = Bundle By Name(cluster=w454, "value"=w453, "sourcePropertyType"=T11."Window behavior") -> (w457:T8)
                n129 = Build Array (concatenate)(w456, w457) -> (w455:T10)
              }
              frame "Allow user to close window" {
                n130 = Bundle By Name(cluster=w461, "value"=w462, "sourcePropertyType"=T11."Allow user to close window") -> (w466:T8)
                n131 = Build Array (concatenate)(w465, w466) -> (w464:T10)
              }
              frame "Window has title bar" {
                n132 = Bundle By Name(cluster=w469, "value"=w467, "sourcePropertyType"=T11."Window has title bar") -> (w472:T8)
                n133 = Build Array (concatenate)(w471, w472) -> (w470:T10)
              }
              frame "Show menu bar" {
                n134 = Bundle By Name(cluster=w475, "value"=w473, "sourcePropertyType"=T11."Show menu bar") -> (w478:T8)
                n135 = Build Array (concatenate)(w477, w478) -> (w476:T10)
              }
              frame "Show tool bar when running" {
                n136 = Bundle By Name(cluster=w479, "value"=w480, "sourcePropertyType"=T11."Show toolbar") -> (w484:T8)
                n137 = Build Array (concatenate)(w483, w484) -> (w482:T10)
              }
              frame "Show scroll bars" {
                n138 = Bundle By Name(cluster=w487, "value"=w485, "sourcePropertyType"=T11."Show vertical scroll bar") -> (w492:T8)
                n139 = Bundle By Name(cluster=w487, "value"=w485, "sourcePropertyType"=T11."Show horizontal scroll bar") -> (w486:T8)
                n140 = Build Array (concatenate)(w491, w492, w486) -> (w490:T10)
              }
              frame "Auto-center" {
                n141 = Select(t=enum16{"Unchanged", "Centered", "Maximized"}."Centered" ("windowRunTimePosition"), s=w501, f=enum16{"Unchanged", "Centered", "Maximized"}."Unchanged" ("windowRunTimePosition")) -> (s? t:f=w495:enum16{"Unchanged", "Centered", "Maximized"})
                n142 = Bundle By Name(cluster=w493, "value"=w495, "sourcePropertyType"=T11."Window run-time position") -> (w498:T8)
                n143 = Build Array (concatenate)(w497, w498) -> (w496:T10)
              }
              frame "Size to entire screen" {
                n144 = Select(t=enum16{"Unchanged", "Centered", "Maximized"}."Maximized" ("windowRunTimePosition"), s=w510, f=enum16{"Unchanged", "Centered", "Maximized"}."Unchanged" ("windowRunTimePosition")) -> (s? t:f=w504:enum16{"Unchanged", "Centered", "Maximized"})
                n145 = Bundle By Name(cluster=w502, "value"=w504, "sourcePropertyType"=T11."Window run-time position") -> (w507:T8)
                n146 = Build Array (concatenate)(w506, w507) -> (w505:T10)
              }
              frame "Automatic error handling" {
                n147 = Bundle By Name(cluster=w513, "value"=w511, "sourcePropertyType"=T11."Auto error handling") -> (w516:T8)
                n148 = Build Array (concatenate)(w515, w516) -> (w514:T10)
              }
            }
          }
          n149 = Equal?(x=w290, y=AB_Source_Inclusion."IncludeIfReferenced" ("sourceInfo.sourceInclusion")) -> (x = y?=w289:bool)
          n150 = Compound Arithmetic op=AND(w289, invert w287, invert w288) -> (w286:bool)
          n151 = Select(t=-1, s=w286, f=w285) -> (s? t:f=w284:i32)
          n152 = call <resource>:"mxLvGetStringProperty.vi"("Tag"=w314, "Item"=w347) -> ("Value"=w346:string, "Item"=w345:T4)  [unwired: 7 in, 1 out]
          n153 = case shown="\"Apply New Password\"" w346 {
            tunnel: w345 -> [_ w394 _]
            tunnel: w313 -> [_ w393 _]
            tunnel: w307 -> [w387 w392 w399]
            tunnel: [w387 w388 w396] -> w344
            frame "No Password Change", Default {
            }
            frame "Apply New Password" {
              n154 = call <resource>:"mxLvGetStringProperty.vi"("Tag"=w393, "Item"=w394) -> ("Value"=w390:string)  [unwired: 7 in, 2 out]
              n155 = Bundle("sourcePropertyType"=T11."Password", "Value"=w390) -> (w389:T14)  [unwired: 1 in]
              n156 = Build Array (concatenate)(w389, w392) -> (w388:T10)
            }
            frame "Remove Password" {
              n157 = Bundle("sourcePropertyType"=T11."Password", "") -> (w397:T15)  [unwired: 1 in]
              n158 = Build Array (concatenate)(w397, w399) -> (w396:T10)
            }
          }
          n159 = Equal?(x=LVFileType."Run-time menu", y=w302) -> (x = y?=w301:bool)
          n160 = Bundle By Name(cluster=w310, "lvfile"=w301, "itemID"=w342, "sourceInclusion"=w290, "destinationIndex"=w284, "properties"=w344) -> (w351:T6)
        }
        frame "writePrevious" {
          # "Containers in < 8.5 (folders and libraries) also saved their item inclusion type. This type is different than the value for folder inclusion. Need to write this so containers appear in the inclusion trees properly."
          # "Libraries were treated as folders and files in 8.2 so need to write Inclusion tag as well as folder tag."
          # "We don't support this in the new code, but need to write it for every item or the setting will be active in old code."
          # "Switching the order of Destination and Support Directories"
          n161 = Unbundle By Name(w549) -> ("buildType"=w534:T2, "folder"=w520:bool, "isLibrary"=w519:bool)
          n162 = Unbundle By Name(w572) -> ("itemID"=w551:string, "sourceInclusion"=w550:T5, "destinationIndex"=w527:i32, "properties"=w533:T10)
          n163 = Build Array(w566, w565) -> (w570:string[])
          n164 = Build Array(w522, w564, w563, w562, w561, w560, w559) -> (w537:string[])
          n165 = Build Array(w558, w557, w556, w555, w554, w553, w552) -> (w538:string[])
          n166 = for {
            tunnel: w523 -> [w625]
            tunnel: w570 -> [w624] mode=indexing
            tunnel: [w623] -> w568 mode=indexing
            n167 = Concatenate Strings(w625, w624) -> (w623:string)
          }
          n168 = Index Array(array=w568) -> (element #1=w546:string, element #2=w545:string)  [unwired: 2 in]
          n169 = case shown="True" w520 {
            selector: w520 -> [_ w594]
            tunnel: [w593 w597] -> w548
            tunnel: w547 -> [w593 w596]
            tunnel: w546 -> [_ w595]
            frame False {
            }
            frame True {
              n170 = call <resource>:"mxLvSetBooleanProperty.vi"("Value (F)"=w594, "Tag"=w595, "Item"=w596) -> ("Item"=w597:T4)  [unwired: 7 in, 1 out]
            }
          }
          n171 = Select(t=w538, s=w520, f=w537) -> (s? t:f=w569:string[])
          n172 = call <resource>:"mxLvSetRefProperty.vi"("Value (\"\")"=w551, "Tag"=w545, "Item"=w548) -> ("Item"=w531:T4)  [unwired: 7 in, 1 out]
          n173 = case shown="\"Include\"" w550 {
            tunnel: w534 -> [_ w602 _ w611]
            tunnel: w520 -> [_ w601 _ w610]
            tunnel: [w598 w600 w607 w609] -> w524
            tunnel: [w598 w599 w607 w608] -> w517
            frame "IncludeIfReferenced" {
              w598 = "As Needed"
            }
            frame "Include" {
              n174 = case shown="\"SourceDist\"" w602 {
                tunnel: w601 -> [_ w606]
                tunnel: [_ w604] -> w600
                tunnel: [_ w603] -> w599
                frame "SourceDist" {
                  (unwired) "Always Include"
                  # "In < 8.5, all items were considered Always Included by default. So returning an empty string which will cause us NOT to write the property. Previous versions will treat a missing property as default."
                }
                frame "EXE", Default {
                  w603 = "Always Included"
                  n175 = Select(t="Dynamic VI (for non-VIs, always include)", s=w606, f=w603) -> (s? t:f=w604:string)
                }
              }
            }
            frame "Exclude" {
              w607 = "Always Exclude"
            }
            frame "TopLevel" {
              n176 = case shown="\"EXE\", Default" w611 {
                tunnel: w610 -> [w615 w619]
                tunnel: [w613 w617] -> w609
                tunnel: [w612 w616] -> w608
                frame "EXE", Default {
                  w612 = "Startup VI"
                  # "\"Include\" is misspelled but that's the way it was. DON'T CORRECT."
                  n177 = Select(t="Top-level VI (for non-VIs, always inclue)", s=w615, f=w612) -> (s? t:f=w613:string)
                }
                frame "DLL" {
                  w616 = "Exported VI"
                  # "\"Include\" is misspelled but that's the way it was. DON'T CORRECT."
                  n178 = Select(t="Top-level VI (for non-VIs, always inclue)", s=w619, f=w616) -> (s? t:f=w617:string)
                }
              }
            }
          }
          n179 = Concatenate Strings(w523, w522) -> (w521:string)
          n180 = Concatenate Strings(w523, "FolderTopLevelVI") -> (w529:string)
          n181 = for {
            tunnel: w523 -> [w622]
            tunnel: w569 -> [w621] mode=indexing
            tunnel: [w620] -> w567 mode=indexing
            n182 = Concatenate Strings(w622, w621) -> (w620:string)
          }
          n183 = call <resource>:"mxLvSetStringProperty.vi"("Value (\"\")"="Never" ("Value (\"\")"), "Tag"=w529, "Item"=w531) -> ("Item"=w530:T4)  [unwired: 7 in, 1 out]
          n184 = Index Array(array=w567) -> (element #1=w544:string, element #2=w543:string, element #3=w542:string, element #4=w541:string, element #5=w540:string, element #6=w536:string, element #7=w535:string)  [unwired: 7 in]
          n185 = case shown="Default" w527 {
            selector: w527 -> [_ w584]
            tunnel: w543 -> [_ w587]
            tunnel: [w583 w586] -> w539
            tunnel: w530 -> [w583 w585]
            frame 0 {
            }
            frame Default {
              n186 = call <resource>:"mxLvSetIntProperty.vi"("Value (0)"=w584, "Tag"=w587, "Item"=w585) -> ("Item"=w586:T4)  [unwired: 7 in, 1 out]
            }
          }
          n187 = case shown="Default" w524 {
            selector: w524 -> [_ w589]
            tunnel: w544 -> [_ w592]
            tunnel: w539 -> [w588 w591]
            tunnel: [w588 w590] -> w526
            frame "" {
            }
            frame Default {
              n188 = call <resource>:"mxLvSetStringProperty.vi"("Value (\"\")"=w589, "Tag"=w592, "Item"=w591) -> ("Item"=w590:T4)  [unwired: 7 in, 1 out]
            }
          }
          n189 = Or(x=w520, y=w519) -> (x .or. y?=w518:bool)
          n190 = case shown="True" w518 {
            tunnel: w526 -> [w573 w577]
            tunnel: [w573 w576] -> w525
            tunnel: w517 -> [_ w575]
            tunnel: w521 -> [_ w574]
            frame False {
            }
            frame True {
              n191 = case shown="Default" w575 {
                selector: w575 -> [_ w579]
                tunnel: w574 -> [_ w582]
                tunnel: w577 -> [w578 w581]
                tunnel: [w578 w580] -> w576
                frame "" {
                }
                frame Default {
                  n192 = call <resource>:"mxLvSetStringProperty.vi"("Value (\"\")"=w579, "Tag"=w582, "Item"=w581) -> ("Item"=w580:T4)  [unwired: 7 in, 1 out]
                }
              }
            }
          }
          n193 = Array Size(array=w533) -> (size(s)=w571:i32)
          n194 = case shown="Default" w571 {
            selector: w571 -> [_ w633]
            tunnel: w533 -> [_ w631]
            tunnel: w542 -> [_ w635]
            tunnel: w525 -> [_ w634]
            tunnel: w541 -> [_ w630]
            tunnel: w540 -> [_ w629]
            tunnel: w536 -> [_ w628]
            tunnel: w535 -> [_ w627]
            tunnel: w534 -> [_ w626]
            frame 0 {
            }
            frame Default {
              n195 = call <resource>:"mxLvSetIntProperty.vi"("Value (0)"=w633, "Tag"=w635, "Item"=w634) -> ("Item"=w632:T4)  [unwired: 7 in, 1 out]
              n196 = for {
                shift-right: [w644] -> _
                shift-left: w632 -> [w640]
                tunnel: w631 -> [w648] mode=indexing
                tunnel: w630 -> [w647]
                tunnel: w629 -> [w646]
                tunnel: w628 -> [w638]
                tunnel: w627 -> [w637]
                tunnel: w626 -> [w636]
                i -> [w645]
                n197 = Unbundle(w648) -> ("sourcePropertyType"=w641:T11, "value"=w642:variant)
                n198 = Format Into String(format string=w647, w645) -> (resulting string=w639:string)  [unwired: 2 in, 1 out]
                n199 = Format Into String(format string=w646, w645) -> (resulting string=w643:string)  [unwired: 2 in, 1 out]
                n200 = case shown="\"Window run-time position\"" w641 {
                  tunnel: w640 -> [w650 w660 w676 w687 w697 w707 w717 w727 w737 w747 w757 w769 w781 w803 w813 w824]
                  tunnel: [w658 w668 w677 w695 w705 w715 w725 w735 w745 w755 w767 w777 w780 w811 w822 w832] -> w644
                  tunnel: w643 -> [w657 w667 _ w694 w704 w714 w724 w734 w744 w754 w766 w776 w778 w810 w821 w831]
                  tunnel: w642 -> [w656 w666 w670 w693 w703 w713 w723 w733 w743 w753 w765 w775 w784 w809 w820 w830]
                  tunnel: w639 -> [w653 w663 _ w690 w700 w710 w720 w730 w740 w750 w764 w772 w779 w806 w817 w828]
                  tunnel: w638 -> [_ _ w669 _ _ _ _ _ _ _ _ _ _ _ _ _]
                  tunnel: w637 -> [_ _ w675 _ _ _ _ _ _ _ _ _ _ _ _ _]
                  tunnel: w636 -> [_ _ w671 _ _ _ _ _ _ _ _ _ _ _ _ _]
                  frame "Remove block diagram" {
                    w652 = T12."Remove diagram"  # old typedef(disconnected)
                    n201 = Format Into String(w652) -> (resulting string=w651:string)  [unwired: 3 in, 1 out]
                    n202 = call <resource>:"mxLvSetStringProperty.vi"("Value (\"\")"=w651, "Tag"=w653, "Item"=w650) -> ("Item"=w649:T4)  [unwired: 7 in, 1 out]
                    n203 = Variant To Data(type=FALSE, Variant=w656) -> (data=w654:bool)  [unwired: 1 in, 1 out]
                    n204 = call <resource>:"mxLvSetBooleanProperty.vi"("Value (F)"=w654, "Tag"=w657, "Item"=w649) -> ("Item"=w658:T4)  [unwired: 7 in, 1 out]
                  }
                  frame "Remove front panel" {
                    w662 = T12."Remove panel"  # old typedef(disconnected)
                    n205 = Format Into String(w662) -> (resulting string=w661:string)  [unwired: 3 in, 1 out]
                    n206 = call <resource>:"mxLvSetStringProperty.vi"("Value (\"\")"=w661, "Tag"=w663, "Item"=w660) -> ("Item"=w659:T4)  [unwired: 7 in, 1 out]
                    n207 = Variant To Data(type=FALSE, Variant=w666) -> (data=w664:bool)  [unwired: 1 in, 1 out]
                    n208 = call <resource>:"mxLvSetBooleanProperty.vi"("Value (F)"=w664, "Tag"=w667, "Item"=w659) -> ("Item"=w668:T4)  [unwired: 7 in, 1 out]
                  }
                  frame "Password" {
                    n209 = case shown="\"SourceDist\"" w671 {
                      tunnel: w670 -> [w681 _]
                      tunnel: [w679 _] -> w674
                      tunnel: [w678 _] -> w673
                      frame "SourceDist" {
                        n210 = Variant To Data(type="", Variant=w681) -> (data=w680:string)  [unwired: 1 in, 1 out]
                        n211 = case shown="Default" w680 {
                          selector: w680 -> [w684 _]
                          tunnel: [w684 "Remove Password"] -> w679
                          tunnel: ["Apply New Password" _] -> w678
                          frame Default {
                          }
                          frame "" {
                          }
                        }
                      }
                      frame Default {
                      }
                    }
                    n212 = call <resource>:"mxLvSetStringProperty.vi"("Value (\"\")"=w674, "Tag"=w669, "Item"=w676) -> ("Item"=w672:T4)  [unwired: 7 in, 1 out]
                    n213 = call <resource>:"mxLvSetStringProperty.vi"("Value (\"\")"=w673, "Tag"=w675, "Item"=w672) -> ("Item"=w677:T4)  [unwired: 7 in, 1 out]
                  }
                  frame "Window has title bar" {
                    w689 = T12."Window has title bar"  # old typedef(disconnected)
                    n214 = Format Into String(w689) -> (resulting string=w688:string)  [unwired: 3 in, 1 out]
                    n215 = call <resource>:"mxLvSetStringProperty.vi"("Value (\"\")"=w688, "Tag"=w690, "Item"=w687) -> ("Item"=w686:T4)  [unwired: 7 in, 1 out]
                    n216 = Variant To Data(type=FALSE, Variant=w693) -> (data=w691:bool)  [unwired: 1 in, 1 out]
                    n217 = call <resource>:"mxLvSetBooleanProperty.vi"("Value (F)"=w691, "Tag"=w694, "Item"=w686) -> ("Item"=w695:T4)  [unwired: 7 in, 1 out]
                  }
                  frame "Show menu bar" {
                    w699 = T12."Show menu bar"  # old typedef(disconnected)
                    n218 = Format Into String(w699) -> (resulting string=w698:string)  [unwired: 3 in, 1 out]
                    n219 = call <resource>:"mxLvSetStringProperty.vi"("Value (\"\")"=w698, "Tag"=w700, "Item"=w697) -> ("Item"=w696:T4)  [unwired: 7 in, 1 out]
                    n220 = Variant To Data(type=FALSE, Variant=w703) -> (data=w701:bool)  [unwired: 1 in, 1 out]
                    n221 = call <resource>:"mxLvSetBooleanProperty.vi"("Value (F)"=w701, "Tag"=w704, "Item"=w696) -> ("Item"=w705:T4)  [unwired: 7 in, 1 out]
                  }
                  frame "Show vertical scroll bar" {
                    w709 = T12."Show scroll bars"  # old typedef(disconnected)
                    n222 = Format Into String(w709) -> (resulting string=w708:string)  [unwired: 3 in, 1 out]
                    n223 = call <resource>:"mxLvSetStringProperty.vi"("Value (\"\")"=w708, "Tag"=w710, "Item"=w707) -> ("Item"=w706:T4)  [unwired: 7 in, 1 out]
                    n224 = Variant To Data(type=FALSE, Variant=w713) -> (data=w711:bool)  [unwired: 1 in, 1 out]
                    n225 = call <resource>:"mxLvSetBooleanProperty.vi"("Value (F)"=w711, "Tag"=w714, "Item"=w706) -> ("Item"=w715:T4)  [unwired: 7 in, 1 out]
                  }
                  frame "Show horizontal scroll bar" {
                    w719 = T12."Show scroll bars"  # old typedef(disconnected)
                    n226 = Format Into String(w719) -> (resulting string=w718:string)  [unwired: 3 in, 1 out]
                    n227 = call <resource>:"mxLvSetStringProperty.vi"("Value (\"\")"=w718, "Tag"=w720, "Item"=w717) -> ("Item"=w716:T4)  [unwired: 7 in, 1 out]
                    n228 = Variant To Data(type=FALSE, Variant=w723) -> (data=w721:bool)  [unwired: 1 in, 1 out]
                    n229 = call <resource>:"mxLvSetBooleanProperty.vi"("Value (F)"=w721, "Tag"=w724, "Item"=w716) -> ("Item"=w725:T4)  [unwired: 7 in, 1 out]
                  }
                  frame "Show toolbar" {
                    w728 = T12."Show tool bar when running"  # old typedef(disconnected)
                    n230 = Format Into String(w728) -> (resulting string=w729:string)  [unwired: 3 in, 1 out]
                    n231 = call <resource>:"mxLvSetStringProperty.vi"("Value (\"\")"=w729, "Tag"=w730, "Item"=w727) -> ("Item"=w726:T4)  [unwired: 7 in, 1 out]
                    n232 = Variant To Data(type=FALSE, Variant=w733) -> (data=w731:bool)  [unwired: 1 in, 1 out]
                    n233 = call <resource>:"mxLvSetBooleanProperty.vi"("Value (F)"=w731, "Tag"=w734, "Item"=w726) -> ("Item"=w735:T4)  [unwired: 7 in, 1 out]
                  }
                  frame "Show Abort button" {
                    w738 = T12."Show abort button"  # old typedef(disconnected)
                    n234 = Format Into String(w738) -> (resulting string=w739:string)  [unwired: 3 in, 1 out]
                    n235 = call <resource>:"mxLvSetStringProperty.vi"("Value (\"\")"=w739, "Tag"=w740, "Item"=w737) -> ("Item"=w736:T4)  [unwired: 7 in, 1 out]
                    n236 = Variant To Data(type=FALSE, Variant=w743) -> (data=w741:bool)  [unwired: 1 in, 1 out]
                    n237 = call <resource>:"mxLvSetBooleanProperty.vi"("Value (F)"=w741, "Tag"=w744, "Item"=w736) -> ("Item"=w745:T4)  [unwired: 7 in, 1 out]
                  }
                  frame "Show fp when called" {
                    w748 = T12."Show panel when called"  # old typedef(disconnected)
                    n238 = Format Into String(w748) -> (resulting string=w749:string)  [unwired: 3 in, 1 out]
                    n239 = call <resource>:"mxLvSetStringProperty.vi"("Value (\"\")"=w749, "Tag"=w750, "Item"=w747) -> ("Item"=w746:T4)  [unwired: 7 in, 1 out]
                    n240 = Variant To Data(type=FALSE, Variant=w753) -> (data=w751:bool)  [unwired: 1 in, 1 out]
                    n241 = call <resource>:"mxLvSetBooleanProperty.vi"("Value (F)"=w751, "Tag"=w754, "Item"=w746) -> ("Item"=w755:T4)  [unwired: 7 in, 1 out]
                  }
                  frame "Window behavior" {
                    w762 = T12."Window is modal"  # old typedef(disconnected)
                    n242 = Format Into String(w762) -> (resulting string=w763:string)  [unwired: 3 in, 1 out]
                    n243 = Variant To Data(type=AB_Source_Property_WindowBehavior."Default" ("windowBehavior"), Variant=w765) -> (data=w760:T9)  [unwired: 1 in, 1 out]
                    n244 = Equal?(x=AB_Source_Property_WindowBehavior."Modal" ("windowBehavior"), y=w760) -> (x = y?=w758:bool)
                    n245 = call <resource>:"mxLvSetStringProperty.vi"("Value (\"\")"=w763, "Tag"=w764, "Item"=w757) -> ("Item"=w756:T4)  [unwired: 7 in, 1 out]
                    n246 = call <resource>:"mxLvSetBooleanProperty.vi"("Value (F)"=w758, "Tag"=w766, "Item"=w756) -> ("Item"=w767:T4)  [unwired: 7 in, 1 out]
                  }
                  frame "Allow user to close window" {
                    w770 = T12."Allow user to close window"  # old typedef(disconnected)
                    n247 = Format Into String(w770) -> (resulting string=w771:string)  [unwired: 3 in, 1 out]
                    n248 = call <resource>:"mxLvSetStringProperty.vi"("Value (\"\")"=w771, "Tag"=w772, "Item"=w769) -> ("Item"=w768:T4)  [unwired: 7 in, 1 out]
                    n249 = Variant To Data(type=FALSE, Variant=w775) -> (data=w773:bool)  [unwired: 1 in, 1 out]
                    n250 = call <resource>:"mxLvSetBooleanProperty.vi"("Value (F)"=w773, "Tag"=w776, "Item"=w768) -> ("Item"=w777:T4)  [unwired: 7 in, 1 out]
                  }
                  frame "Window run-time position" {
                    n251 = Variant To Data(type=enum16{"Unchanged", "Centered", "Maximized"}."Unchanged" ("windowRunTimePosition"), Variant=w784) -> (data=w782:enum16{"Unchanged", "Centered", "Maximized"})  [unwired: 1 in, 1 out]
                    n252 = case shown="\"Centered\"" w782 {
                      tunnel: w781 -> [w785 w793 w801]
                      tunnel: [w785 w792 w800] -> w780
                      tunnel: w779 -> [_ w787 w795]
                      tunnel: w778 -> [_ w786 w794]
                      frame Default {
                      }
                      frame "Centered" {
                        n253 = Format Into String(T12."Auto-center" ("old typedef(disconnected)")) -> (resulting string=w788:string)  [unwired: 3 in, 1 out]
                        n254 = call <resource>:"mxLvSetStringProperty.vi"("Value (\"\")"=w788, "Tag"=w787, "Item"=w793) -> ("Item"=w790:T4)  [unwired: 7 in, 1 out]
                        n255 = call <resource>:"mxLvSetBooleanProperty.vi"("Value (F)"=TRUE, "Tag"=w786, "Item"=w790) -> ("Item"=w792:T4)  [unwired: 7 in, 1 out]
                      }
                      frame "Maximized" {
                        n256 = Format Into String(T12."Size to entire screen" ("old typedef(disconnected)")) -> (resulting string=w796:string)  [unwired: 3 in, 1 out]
                        n257 = call <resource>:"mxLvSetStringProperty.vi"("Value (\"\")"=w796, "Tag"=w795, "Item"=w801) -> ("Item"=w798:T4)  [unwired: 7 in, 1 out]
                        n258 = call <resource>:"mxLvSetBooleanProperty.vi"("Value (F)"=TRUE, "Tag"=w794, "Item"=w798) -> ("Item"=w800:T4)  [unwired: 7 in, 1 out]
                      }
                    }
                  }
                  frame "Run when opened" {
                    w804 = T12."Run when opened"  # old typedef(disconnected)
                    n259 = Format Into String(w804) -> (resulting string=w805:string)  [unwired: 3 in, 1 out]
                    n260 = call <resource>:"mxLvSetStringProperty.vi"("Value (\"\")"=w805, "Tag"=w806, "Item"=w803) -> ("Item"=w802:T4)  [unwired: 7 in, 1 out]
                    n261 = Variant To Data(type=FALSE, Variant=w809) -> (data=w807:bool)  [unwired: 1 in, 1 out]
                    n262 = call <resource>:"mxLvSetBooleanProperty.vi"("Value (F)"=w807, "Tag"=w810, "Item"=w802) -> ("Item"=w811:T4)  [unwired: 7 in, 1 out]
                  }
                  frame "Allow debugging" {
                    w815 = T12."Remove debugging"  # old typedef(disconnected)
                    n263 = Format Into String(w815) -> (resulting string=w816:string)  [unwired: 3 in, 1 out]
                    n264 = Variant To Data(type=FALSE, Variant=w820) -> (data=w818:bool)  [unwired: 1 in, 1 out]
                    n265 = call <resource>:"mxLvSetStringProperty.vi"("Value (\"\")"=w816, "Tag"=w817, "Item"=w813) -> ("Item"=w812:T4)  [unwired: 7 in, 1 out]
                    n266 = Not(x=w818) -> (.not. x?=w814:bool)
                    n267 = call <resource>:"mxLvSetBooleanProperty.vi"("Value (F)"=w814, "Tag"=w821, "Item"=w812) -> ("Item"=w822:T4)  [unwired: 7 in, 1 out]
                  }
                  frame "Auto error handling" {
                    w826 = T12."Automatic error handling"  # old typedef(disconnected)
                    n268 = Format Into String(w826) -> (resulting string=w827:string)  [unwired: 3 in, 1 out]
                    n269 = call <resource>:"mxLvSetStringProperty.vi"("Value (\"\")"=w827, "Tag"=w828, "Item"=w824) -> ("Item"=w823:T4)  [unwired: 7 in, 1 out]
                    n270 = Variant To Data(type=FALSE, Variant=w830) -> (data=w825:bool)  [unwired: 1 in, 1 out]
                    n271 = call <resource>:"mxLvSetBooleanProperty.vi"("Value (F)"=w825, "Tag"=w831, "Item"=w823) -> ("Item"=w832:T4)  [unwired: 7 in, 1 out]
                  }
                }
              }
            }
          }
        }
        frame "clearPrevious" {
          n272 = Build Array(w846, w847, w875, w874, w862, w873, w872) -> (w849:string[])
          n273 = Build Array(w871, w870, w859, w869, w868) -> (w845:string[])
          n274 = Concatenate Strings(w854, w862) -> (w863:string)
          n275 = Concatenate Strings(w854, w861) -> (w860:string)
          n276 = Concatenate Strings(w854, w858) -> (w857:string)
          n277 = Concatenate Strings(w854, w859) -> (w853:string)
          n278 = Concatenate Strings(w854, w856) -> (w852:string)
          n279 = Concatenate Strings(w854, w855) -> (w851:string)
          n280 = call <resource>:"mxLvGetIntProperty.vi"("Tag"=w863, "Item"=w865) -> ("Value"=w867:i32, "Item"=w866:T4)  [unwired: 7 in, 1 out]
          n281 = for {
            N: w867 -> [_]
            tunnel: w860 -> [w887]
            shift-right: [w882] -> w864
            shift-left: w866 -> [w884]
            tunnel: w857 -> [w885]
            i -> [w886]
            n282 = Format Into String(format string=w887, w886) -> (resulting string=w881:string)  [unwired: 2 in, 1 out]
            n283 = Format Into String(format string=w885, w886) -> (resulting string=w880:string)  [unwired: 2 in, 1 out]
            n284 = call <resource>:"mxLvDeleteProperty.vi"("Tag"=w881, "Item"=w884) -> ("Item"=w883:T4)  [unwired: 8 in, 1 out]
            n285 = call <resource>:"mxLvDeleteProperty.vi"("Tag"=w880, "Item"=w883) -> ("Item"=w882:T4)  [unwired: 8 in, 1 out]
          }
          n286 = Build Array("ApplyInclusion", "DisableInclusion", "ApplyDestination", "DisableDestination", "ApplyProperties", "DisableProperties", "ApplyPassword", "DisablePassword", "TopLevelVI", "FolderTopLevelVI", "FolderMask") -> (w833:string[])
          n287 = Build Array (concatenate)(w849, w845, w833) -> (w850:string[])
          n288 = call <resource>:"mxLvGetIntProperty.vi"("Tag"=w853, "Item"=w864) -> ("Value"=w877:i32, "Item"=w878:T4)  [unwired: 7 in, 1 out]
          n289 = for {
            N: w877 -> [_]
            tunnel: w852 -> [w900]
            shift-right: [w895] -> w876
            shift-left: w878 -> [w897]
            tunnel: w851 -> [w898]
            i -> [w899]
            n290 = Format Into String(format string=w900, w899) -> (resulting string=w894:string)  [unwired: 2 in, 1 out]
            n291 = Format Into String(format string=w898, w899) -> (resulting string=w893:string)  [unwired: 2 in, 1 out]
            n292 = call <resource>:"mxLvDeleteProperty.vi"("Tag"=w894, "Item"=w897) -> ("Item"=w896:T4)  [unwired: 8 in, 1 out]
            n293 = call <resource>:"mxLvDeleteProperty.vi"("Tag"=w893, "Item"=w896) -> ("Item"=w895:T4)  [unwired: 8 in, 1 out]
          }
          n294 = for {
            tunnel: w854 -> [w890]
            tunnel: w850 -> [w889] mode=indexing
            tunnel: [w888] -> w848 mode=indexing
            n295 = Concatenate Strings(w890, w889) -> (w888:string)
          }
          n296 = for {
            tunnel: w876 -> [w892]
            tunnel: w848 -> [w891] mode=indexing
            n297 = call <resource>:"mxLvDeleteProperty.vi"("Tag"=w891, "Item"=w892) -> ()  [unwired: 8 in, 2 out]
          }
        }
      }
    }
    frame Error {
    }
  }
  "dataSource out" <- w28
  "error out" <- "error in (no error)"
  "buildObject out" <- "buildObject"
  "index out" <- "index in"
